vi "ReadMessages.vi"(8 "error in (no error)":errorcluster, 10 "NumOfMessages":i32=40, 11 "GPS in":refnum<class "GPS.lvclass">) -> (0 "error out":errorcluster, 2 "Data":string, 3 "GPS out":refnum<class "GPS.lvclass">)   [LabVIEW 2020, in "GPS.lvlib" / "GPS.lvclass"]
uses:
  GPS.lvclass
  C:/Users/dzoni/Documents/NJ/Playground/LV/TCP GPS/lv_tcp_gps/TCP/TCP.lvclass
  GPS.lvclass/GPS.ctl
  TCP/TCP.lvclass/TCP.ctl
  TCP/TCP.lvclass
panel:
  out "NumOfMessagesRead":i32
  out "MessageLengthMin":i32
  out "MessageLengthMax":i32
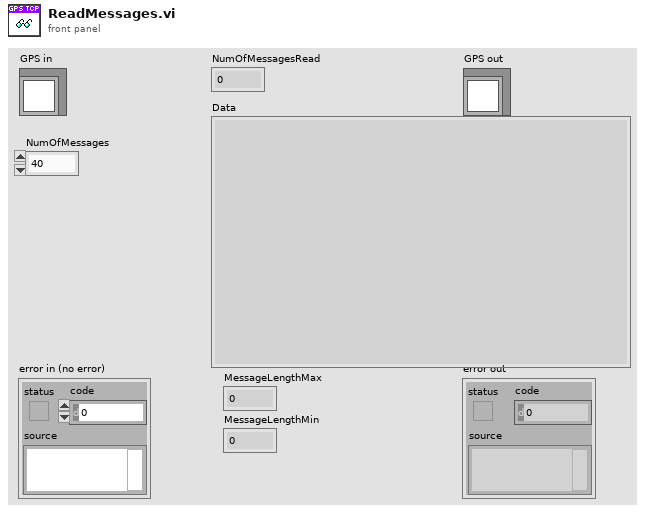
[diagram p1: front panel]
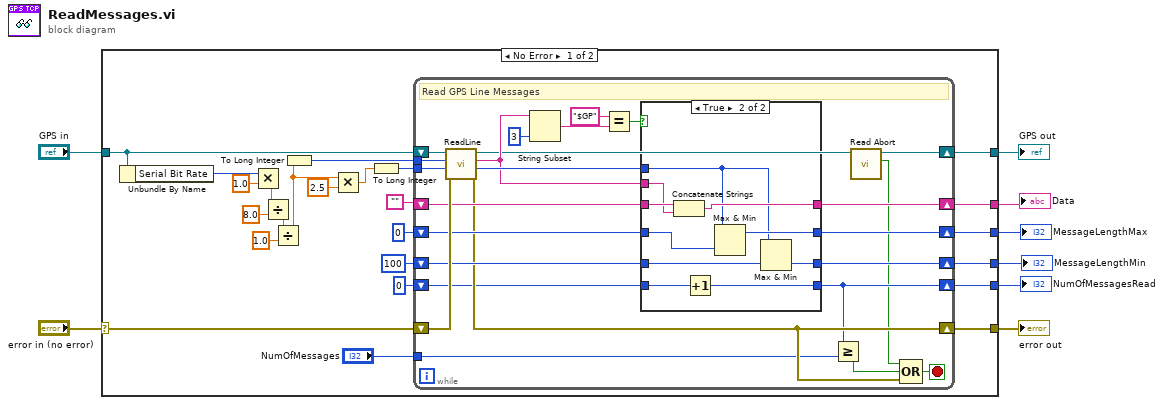
[diagram p0: block diagram]
diagram:
  n1 = case shown="No Error" "error in (no error)" {
    selector: "error in (no error)" -> [w32 w73]
    tunnel: [w31 w73] -> w7
    tunnel: [w29 w72] -> w5
    tunnel: "GPS in" -> [w28 w72]
    tunnel: [w30 _] -> w4
    tunnel: [w20 _] -> w3
    tunnel: [w18 _] -> w2
    tunnel: [w12 _] -> w1
    frame No Error {
      n2 = Unbundle By Name(w28) -> ("Serial Bit Rate"=w27:u32)
      n3 = Multiply(x=w27, y=1.0) -> (x*y=w26:dbl)
      n4 = Divide(x=w26, y=8.0) -> (x/y=w16:dbl)
      n5 = Divide(x=w16, y=1.0) -> (x/y=w10:dbl)
      n6 = To Long Integer(number=w10) -> (32bit integer=w23:i32)
      n7 = Multiply(x=w10, y=2.5) -> (x*y=w24:dbl)
      n8 = To Long Integer(number=w24) -> (32bit integer=w9:i32)
      n9 = while {
        tunnel: w9 -> [w55]
        tunnel: w23 -> [w54]
        shift-right: [w41] -> w31
        shift-left: w32 -> [w57]
        shift-right: [w33] -> w29
        shift-left: w28 -> [w56]
        shift-right: [w53] -> w30
        shift-left: "" -> [w52]
        shift-right: [w50] -> w20
        shift-left: 0 ("Length") -> [w51]
        shift-right: [w49] -> w18
        shift-left: 100 -> [w48]
        shift-right: [w38] -> w12
        shift-left: 0 ("Length") -> [w39]
        tunnel: "NumOfMessages" -> [w37]
        stop <- w40 stop-if-true
        # "Read GPS Line Messages"
        n10 = call-dynamic "ReadLine.vi"("error in (no error)"=w57, "Timeout"=w55, "NumOfBytes"=w54, "ClientBase in"=w56) -> ("error out"=w41:errorcluster, "Length"=w47:i32, "Data"=w46:string, "ClientBase out"=w34:refnum<class "GPS.lvclass">)  [unwired: 4 in]
        n11 = String Subset(string=w46, length (rest)=3 ("length (rest)")) -> (substring=w44:string)  [unwired: 1 in]
        n12 = Equal?(x="$GP", y=w44) -> (x = y?=w42:bool)
        n13 = case shown="True" w42 {
          tunnel: [w61 w71] -> w53
          tunnel: w52 -> [w61 w70]
          tunnel: w51 -> [w60 w69]
          tunnel: [w60 w68] -> w50
          tunnel: [w59 w67] -> w49
          tunnel: w48 -> [w59 w66]
          tunnel: w47 -> [_ w65]
          tunnel: w46 -> [_ w64]
          tunnel: [w58 w63] -> w38
          tunnel: w39 -> [w58 w62]
          frame False {
          }
          frame True {
            n14 = Concatenate Strings(w70, w64) -> (w71:string)
            n15 = Increment(x=w62) -> (x+1=w63:i32)
            n16 = Max & Min(x=w65, y=w69) -> (max(x,y)=w68:i32)  [unwired: 1 out]
            n17 = Max & Min(x=w65, y=w66) -> (min(x,y)=w67:i32)  [unwired: 1 out]
          }
        }
        n18 = Greater Or Equal?(x=w38, y=w37) -> (x >= y?=w36:bool)
        n19 = call "Read Abort.vi"("ClientBase in"=w34) -> ("Abort"=w35:bool, "ClientBase out"=w33:refnum<class "GPS.lvclass">)  [unwired: 8 in, 1 out]
        n20 = Compound Arithmetic op=OR(w35, w36, w41) -> (w40:bool)
      }
    }
    frame Error {
    }
  }
  "error out" <- w7
  "GPS out" <- w5
  "Data" <- w4
  "MessageLengthMax" <- w3
  "MessageLengthMin" <- w2
  "NumOfMessagesRead" <- w1
